vi "Tutorial3_fomula method_TP059851.vi"() -> ()   [LabVIEW 2020]
uses:
  <vilib>/express/express arith-compare/Formula/XNode/ExpressFormulaBlockNode.xnode
panel:
  in  "UI":enum32{"Question1", "question 2"}(tab)
  out "V M1  3":dbl
  out "V M1  2":dbl
  out "V M1":dbl
  out "SA M3":dbl
  out "SA M2":dbl
  out "SA M1":dbl
  in  "Height":dbl
  in  "Radius":dbl
  out "M3":dbl
  out "M2":dbl
  out "M1":dbl
  in  "Y":dbl
  in  "X":dbl
  # "Input"
  # "Surface area"
  # "Volume"
  # "2xy^2 +4xy +8"
  # "Input"
  # "Answer"
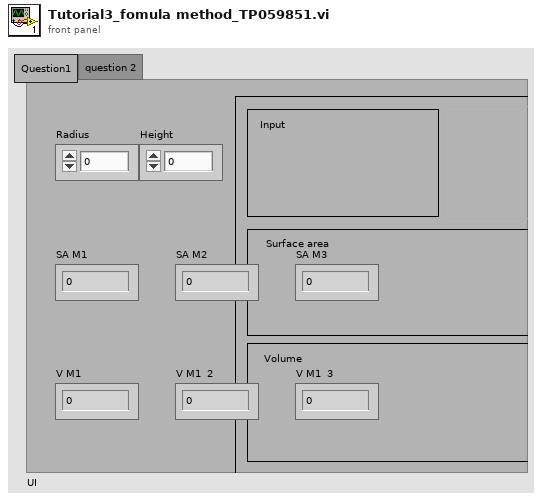
[diagram p1: front panel]
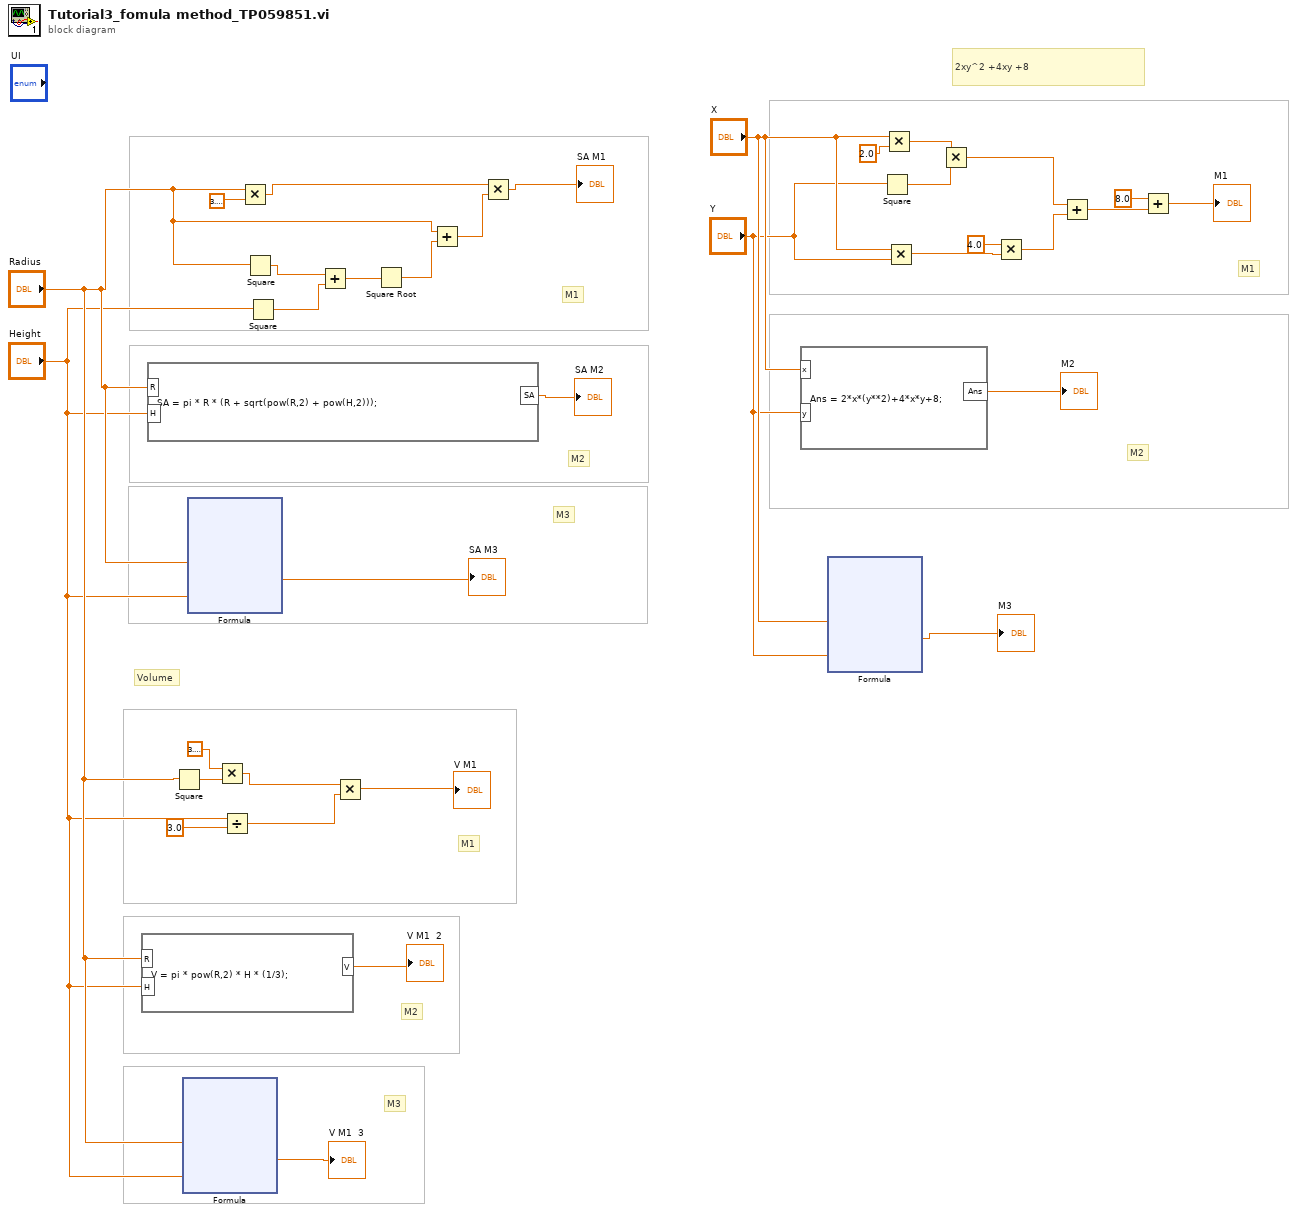
[diagram p0: block diagram]
diagram:
  # "M2"
  # "M1"
  # "2xy^2 +4xy +8"
  # "M3"
  # "M2"
  # "Volume"
  # "M1"
  # "M3"
  # "M2"
  # "SA = pi * R * (R + sqrt(H**2 + R**2)); also can"
  # "M1"
  n1 = formula code="V = pi * pow(R,2) * H * (1/3);"("R"="Radius", "H"="Height") -> ("V"=→"V M1  2":dbl)
  n2 = formula code="SA = pi * R * (R + sqrt(pow(R,2) + pow(H,2)));"("R"="Radius", "H"="Height") -> ("SA"=→"SA M2":dbl)
  n3 = Square(x="Radius") -> (x^2=w23:dbl)
  n4 = xnode "Formula"("R"="Radius", "H"="Height") -> ("Result"=→"V M1  3":dbl)  [unwired: 1 in, 1 out]
  n5 = xnode "Formula"("R"="Radius", "H"="Height") -> ("Result"=→"SA M3":dbl)  [unwired: 1 in, 1 out]
  n6 = Multiply(x=3.141592653589793, y=w23) -> (x*y=w21:dbl)
  n7 = Divide(x="Height", y=3.0) -> (x/y=w20:dbl)
  n8 = Multiply(x="Radius", y=3.141592653589793) -> (x*y=w29:dbl)
  n9 = Square(x="Radius") -> (x^2=w33:dbl)
  n10 = Square(x="Height") -> (x^2=w32:dbl)
  n11 = Add(x=w33, y=w32) -> (x+y=w31:dbl)
  n12 = Multiply(x=w21, y=w20) -> (x*y=→"V M1":dbl)
  n13 = Square Root(x=w31) -> (sqrt(x)=w30:dbl)
  n14 = Add(x="Radius", y=w30) -> (x+y=w28:dbl)
  n15 = Multiply(x=w29, y=w28) -> (x*y=→"SA M1":dbl)
  n16 = formula code="Ans = 2*x*(y**2)+4*x*y+8;"("x"="X", "y"="Y") -> ("Ans"=→"M2":dbl)
  n17 = xnode "Formula"("x"="X", "y"="Y") -> ("Result"=→"M3":dbl)  [unwired: 1 in, 1 out]
  n18 = Square(x="Y") -> (x^2=w7:dbl)
  n19 = Multiply(x="X", y=2.0) -> (x*y=w8:dbl)
  n20 = Multiply(x="X", y="Y") -> (x*y=w6:dbl)
  n21 = Multiply(x=w8, y=w7) -> (x*y=w5:dbl)
  n22 = Multiply(x=4.0, y=w6) -> (x*y=w13:dbl)
  n23 = Add(x=w5, y=w13) -> (x+y=w12:dbl)
  n24 = Add(x=8.0, y=w12) -> (x+y=→"M1":dbl)
